vi "Scan_ver2_2_test.vi"(0 "DMM ref":refnum<visa-resource-name>, 1 "output cluster":cluster{"y":i32, i32, "Sample number":i32}={"y"=0, 0, "Sample number"=1}, 2 "P_current_count":i32, 3 "N_current_count":i32, 5 "DMM error":errorcluster, 7 "Current Sense \nResitance Array":dbl[](array[numeric])=[1.0032214, 1.00250644, 1.00234822, 1.0040944, 1.0017711, 1.00229431, 1.00344206, 1.00482066, 1.00381056, 1.00290978, 1.00333016, 1.00367587], 9 "ESP32 ref":refnum<visa-resource-name>, 11 "ESP32 error":errorcluster, 12 "current_mode":u8[](array[numeric])=[0, 0, 0, 0, 0, 0, 0, 0, 0, 0, 0]) -> (4 "DMM ref":refnum<visa-resource-name>, 6 "DMM error":errorcluster, 8 "Measurements":dbl[](array[numeric]), 10 "ESP32 ref":refnum<visa-resource-name>, 13 "Timout?":bool, 14 "Numeric":u32, 15 "ESP32 error":errorcluster)   [LabVIEW 2023]
uses:
  <instrlib>/Agilent 3446X Series/Agilent 3446X Series.lvlib
panel:
  out "read buffer":string
  out "error out":errorcluster
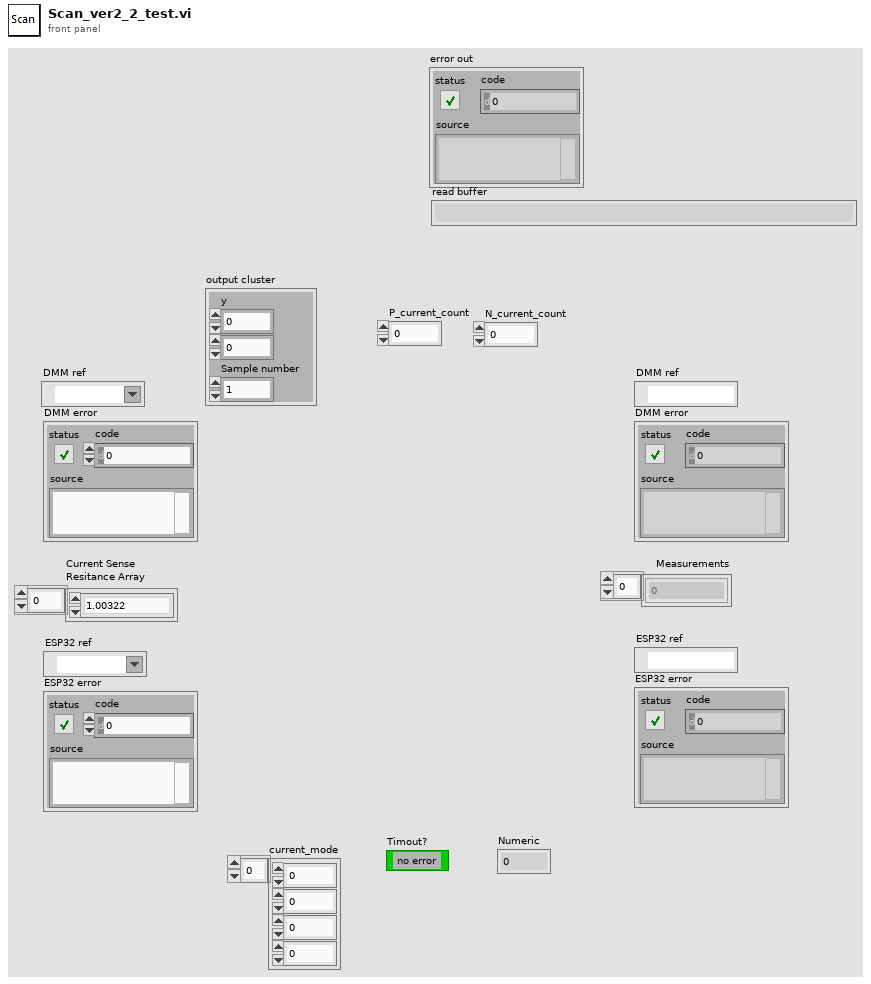
[diagram p1: front panel]
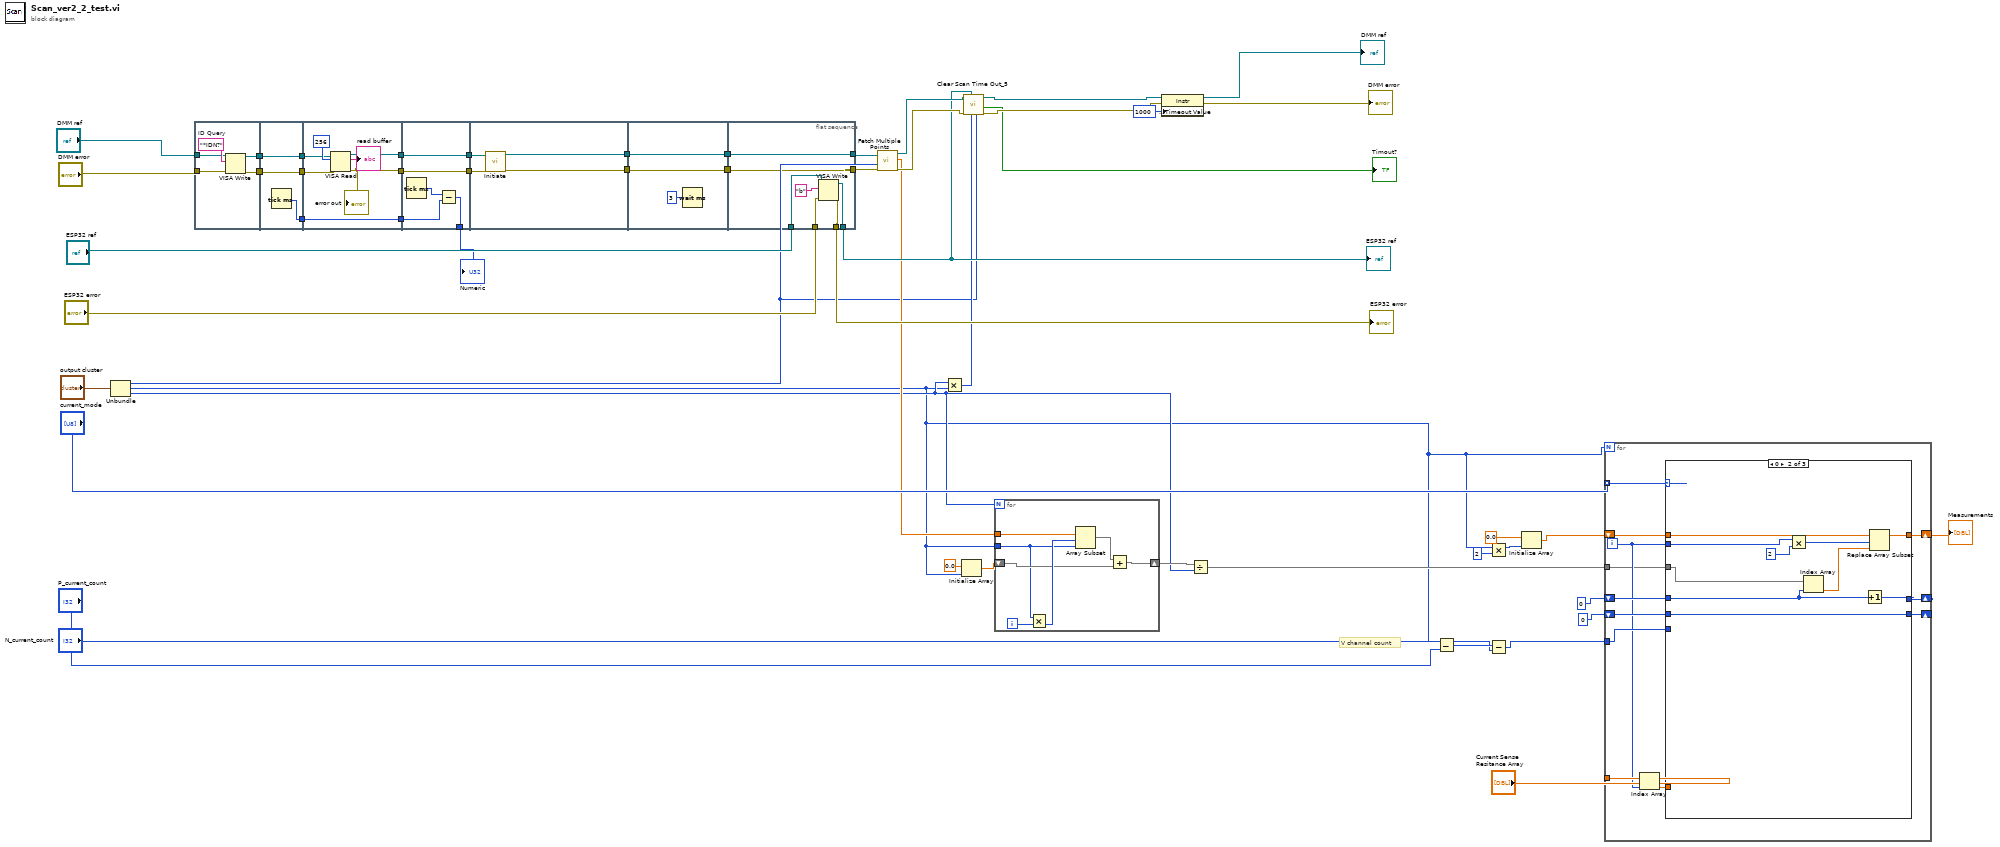
[diagram p0: block diagram]
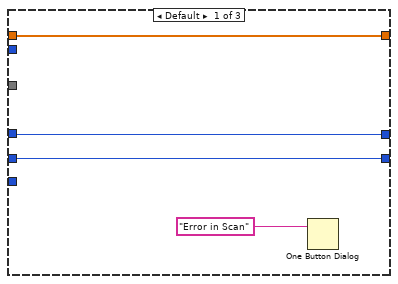
[diagram p2: hidden frame]
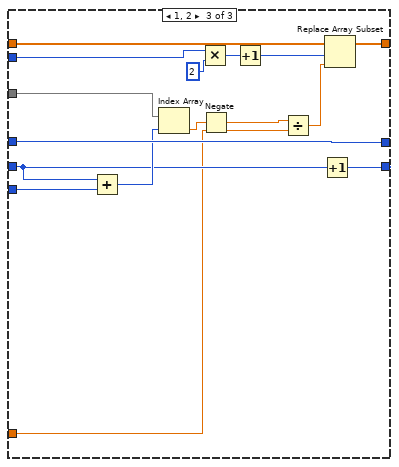
[diagram p3: hidden frame]
diagram:
  # "V channel count"
  n1 = Unbundle("output cluster") -> ("y"=w12:i32, w13:i32, "Sample number"=w14:i32)
  n2 = flat-sequence {
    tunnel: "DMM error" -> [w57]
    tunnel: "DMM ref" -> [w58]
    tunnel: [w56] -> w6
    tunnel: [w55] -> w4
    tunnel: [w62] -> w7
    tunnel: w6 -> [w62]
    tunnel: [w61] -> w5
    tunnel: w4 -> [w61]
    tunnel: [w60] -> w3
    tunnel: [w66] -> w11
    tunnel: [w65] -> w9
    tunnel: w7 -> [w68]
    tunnel: w5 -> [w67]
    tunnel: w3 -> [w64]
    tunnel: [w64] -> w2
    tunnel: w11 -> [w74]
    tunnel: [w74] -> w10
    tunnel: w9 -> [w73]
    tunnel: [w73] -> w8
    tunnel: w2 -> [w71]
    tunnel: [w70] -> w1
    tunnel: [w78] -> w54
    tunnel: [w77] -> w53
    tunnel: w10 -> [w76]
    tunnel: w8 -> [w75]
    tunnel: w54 -> [w81]
    tunnel: [w81] -> w52
    tunnel: w53 -> [w80]
    tunnel: [w80] -> w51
    tunnel: w52 -> [w88]
    tunnel: w51 -> [w87]
    tunnel: "ESP32 ref" -> [w86]
    tunnel: "ESP32 error" -> [w85]
    tunnel: [w84] -> w40
    tunnel: [w83] -> w41
    tunnel: [w88] -> w24
    tunnel: [w87] -> w23
    frame #0 {
      w59 = "*IDN?"  # ID Query
      n3 = VISA Write(VISA resource name=w58, write buffer=w59, error in (no error)=w57) -> (VISA resource name out=w56:refnum<visa-resource-name>, error out=w55:errorcluster)  [unwired: 1 out]
    }
    frame #1 {
      n4 = Tick Count (ms)() -> (millisecond timer value=w60:u32)
    }
    frame #2 {
      n5 = VISA Read(VISA resource name=w68, byte count=u32 256, error in (no error)=w67) -> (VISA resource name out=w66:refnum<visa-resource-name>, read buffer=→"read buffer":string, error out=w65:errorcluster)  [unwired: 1 out]
      "error out" <- w65
    }
    frame #3 {
      n6 = Tick Count (ms)() -> (millisecond timer value=w72:u32)
      n7 = Subtract(x=w72, y=w71) -> (x-y=w70:u32)
    }
    frame #4 {
      n8 = call <instrlib>:"Initiate.vi"("error in (no error)"=w75, "VISA resource name"=w76) -> ("error out"=w78:errorcluster, "VISA resource name out"=w77:refnum<visa-resource-name>)  [unwired: 8 in]
    }
    frame #5 {
      n9 = Wait (ms)(milliseconds to wait=u32 3) -> ()  [unwired: 1 out]
    }
    frame #6 {
      n10 = VISA Write(VISA resource name=w86, write buffer="b" ("data in"), error in (no error)=w85) -> (VISA resource name out=w84:refnum<visa-resource-name>, error out=w83:errorcluster)  [unwired: 1 out]
    }
  }
  n11 = call <instrlib>:"Fetch Multiple Points.vi"("error in (no error)"=w24, "Timeout (10000 ms)"=w12, "VISA resource name"=w23) -> ("error out"=w48:errorcluster, "Measurements"=w19:dbl[], "VISA resource name out"=w49:refnum<visa-resource-name>)  [unwired: 1 in, 5 out]
  n12 = Multiply(x=w14, y=w13) -> (x*y=w15:i32)
  n13 = Initialize Array(0.0 ("element"), w13) -> (w18:dbl[])
  n14 = call "Clear Scan Time Out_5.vi"("Timeout"=w12, "Channel number"=w15, "ESP32 ref"=w40, "error in (no error)"=w48, "VISA Refnum in"=w49) -> ("error out"=w46:errorcluster, "error?"=→"Timout?":bool, "VISA Refnum out"=w47:refnum<visa-resource-name>)  [unwired: 2 in, 2 out]
  n15 = for {
    N: w14 -> [_]
    tunnel: w19 -> [w93]
    shift-right: [w90] -> w17
    shift-left: w18 -> [w91]
    tunnel: w13 -> [w89]
    i -> [w95]
    n16 = Multiply(x=w89, y=w95) -> (x*y=w94:i32)
    n17 = Array Subset(array=w93, index=w94, length=w89) -> (w92:dbl[])
    n18 = Add(x=w92, y=w91) -> (x+y=w90:dbl[])
  }
  n19 = property class="Instr"(reference=w47, error in=w46, "General Settings:Timeout Value"=u32 1000) -> (reference out=→"DMM ref":refnum<visa-resource-name>, error out=→"DMM error":errorcluster)
  n20 = Divide(x=w17, y=w14) -> (x/y=w16:dbl[])
  n21 = Subtract(x=w13, y="P_current_count") -> (x-y=w33:i32)
  n22 = Multiply(x=w13, y=2) -> (x*y=w37:i32)
  n23 = Subtract(x=w33, y="N_current_count") -> (x-y=w21:i32)
  n24 = Initialize Array(0.0 ("Measurement"), w37) -> (w35:dbl[])
  n25 = for {
    N: w13 -> [_]
    shift-right: [w103] -> w28
    shift-left: w35 -> [w104]
    tunnel: "current_mode" -> [w107] mode=indexing
    tunnel: w21 -> [w100]
    shift-right: [w105] -> _
    shift-left: 0 ("index") -> [w106]
    shift-right: [w101] -> _
    shift-left: 0 ("index") -> [w102]
    tunnel: "Current Sense \nResitance Array" -> [w99]
    tunnel: w16 -> [w96]
    i -> [w98]
    n26 = Index Array(array=w99, index=w98) -> (element=w97:dbl)
    n27 = case shown="0" w107 {
      tunnel: w106 -> [w111 w121 w131]
      tunnel: [w111 w120 w131] -> w105
      tunnel: w98 -> [_ w118 w136]
      tunnel: w104 -> [w110 w119 w137]
      tunnel: [w110 w116 w133] -> w103
      tunnel: w102 -> [w109 w115 w128]
      tunnel: [w109 w115 w127] -> w101
      tunnel: w100 -> [_ _ w130]
      tunnel: w97 -> [_ _ w125]
      tunnel: w96 -> [_ w113 w123]
      frame Default {
        n28 = One Button Dialog(message="Error in Scan") -> ()  [unwired: 1 in, 1 out]
      }
      frame 0 {
        n29 = Multiply(x=w118, y=2 ("x")) -> (x*y=w114:i32)
        n30 = Index Array(array=w113, index=w121) -> (element=w112:dbl)
        n31 = Increment(x=w121) -> (x+1=w120:i32)
        n32 = Replace Array Subset(array=w119, new element=w112, index=w114) -> (w116:dbl[])
      }
      frame 1, 2 {
        n33 = Add(x=w128, y=w130) -> (x+y=w129:i32)
        n34 = Index Array(array=w123, index=w129) -> (element=w122:dbl)
        n35 = Multiply(x=w136, y=2 ("x")) -> (x*y=w134:i32)
        n36 = Negate(x=w122) -> (-x=w124:dbl)
        n37 = Increment(x=w134) -> (x+1=w132:i32)
        n38 = Divide(x=w124, y=w125) -> (x/y=w126:dbl)
        n39 = Increment(x=w128) -> (x+1=w127:i32)
        n40 = Replace Array Subset(array=w137, new element=w126, index=w132) -> (w133:dbl[])
      }
    }
  }
  "Measurements" <- w28
  "ESP32 ref" <- w40
  "ESP32 error" <- w41
  "Numeric" <- w1
